vi "Cast to Interfaceable.vi"(2 "Target Object":refnum<class "Interfaceable.lvclass">, 3 "Interface":refnum<class "IUnknown.lvclass">, 4 "error in (no error)":errorcluster) -> (0 "Interfaceable Object":refnum<class "Interfaceable.lvclass">, 1 "error out":errorcluster)   [LabVIEW 2009, in "Interfaceable.lvclass"]
doc: "Casts a concrete interface into the original Interfaceable Object. \n\nWhen an interface has been used to modify by-val properties of an object, use this vi to recover the original object. This vi raises error 510202 if the cast fails."
uses:
  Interfaceable.lvclass
  IUnknown Class/IUnknown.lvclass
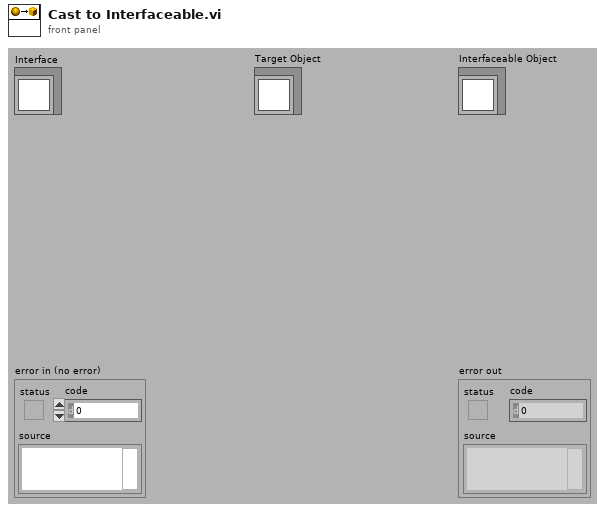
[diagram p1: front panel]
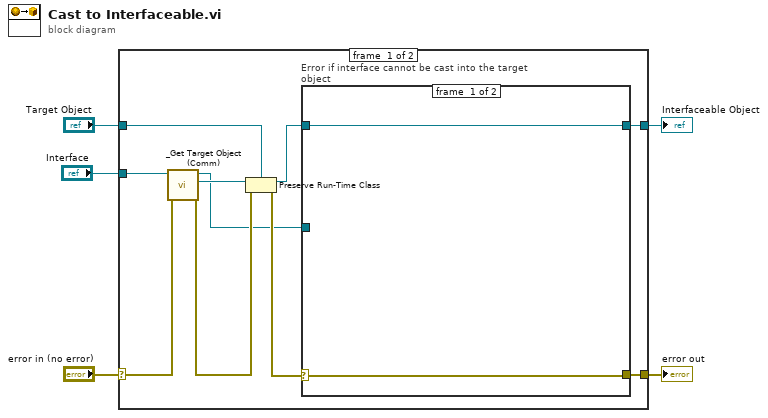
[diagram p0: block diagram]
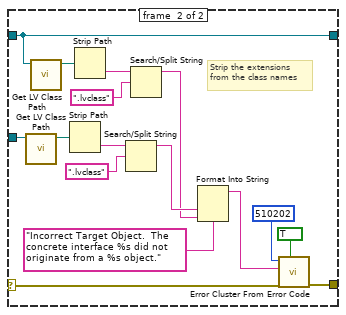
[diagram p2: hidden frame]
diagram:
  n1 = case shown="No Error" "error in (no error)" {
    selector: "error in (no error)" -> [w12 w35]
    tunnel: [w10 w35] -> w4
    tunnel: [w7 w34] -> w2
    tunnel: "Target Object" -> [w13 w34]
    tunnel: "Interface" -> [w15 _]
    frame #0 {
      n2 = call "_Get Target Object (Comm).vi"("error in (no error)"=w12, "Interface in"=w15) -> ("error out"=w11:errorcluster, "Target Object"=w14:refnum<class "Interfaceable.lvclass">, "Interface out"=w6:refnum<class "IUnknown.lvclass">)  [unwired: 7 in]
      n3 = Preserve Run-Time Class(object in=w14, error in=w11, 2:w13) -> (object out=w8:refnum<class "Interfaceable.lvclass">, error out=w9:errorcluster)
      n4 = case "Error if interface cannot be cast into the target object" shown="Error" w9 {
        selector: w9 -> [w17 w31]
        tunnel: [w17 w33] -> w10
        tunnel: [w16 w22] -> w7
        tunnel: w8 -> [w16 w22]
        tunnel: w6 -> [_ w21]
        frame #0 {
        }
        frame #1 {
          # "Strip the extensions from the class names"
          n5 = call <vilib>:"Get LV Class Path.vi"("object"=w21) -> ("class path"=w23:path)  [unwired: 9 in, 1 out]
          n6 = call <vilib>:"Get LV Class Path.vi"("object"=w22) -> ("class path"=w29:path)  [unwired: 9 in, 1 out]
          n7 = Strip Path(path=w23) -> (name=w24:string)  [unwired: 1 out]
          n8 = Strip Path(path=w29) -> (name=w28:string)  [unwired: 1 out]
          n9 = Search/Split String(string=w24, search string/char (-)=".lvclass") -> (substring before match=w26:string)  [unwired: 1 in, 2 out]
          n10 = Search/Split String(string=w28, search string/char (-)=".lvclass") -> (substring before match=w20:string)  [unwired: 1 in, 2 out]
          n11 = Format Into String(format string="Incorrect Target Object.  The concrete interface %s did not originate from a %s object." ("error message (\"\")"), w26, w20) -> (resulting string=w18:string)  [unwired: 2 in, 1 out]
          n12 = call <vilib>:"Error Cluster From Error Code.vi"("show call chain? (False)"=TRUE, "error in (no error)"=w31, "error message (\"\")"=w18, "error code (0)"=510202) -> ("error out"=w33:errorcluster)  [unwired: 5 in]
        }
      }
    }
    frame #1 {
    }
  }
  "error out" <- w4
  "Interfaceable Object" <- w2
